vi "New File.vi"(8 "error in (no error)":errorcluster, 11 "Log in":refnum<class "Log.lvclass">) -> (0 "error out":errorcluster, 3 "Log out":refnum<class "Log.lvclass">)   [LabVIEW 2020, in "Log.lvclass"]
doc: "Starts a new file. Increments the file count, resets the line count and writes the header information into the file."
uses:
  Log.lvclass
  Log.lvclass/Log.ctl
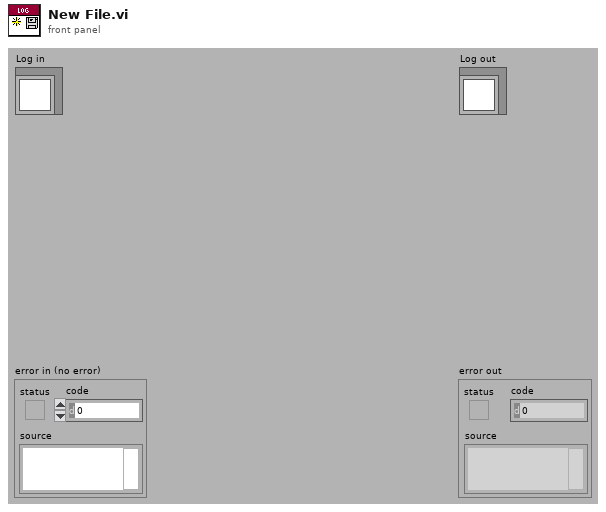
[diagram p1: front panel]
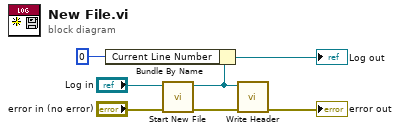
[diagram p0: block diagram]
diagram:
  n1 = call "Start New File.vi"("error in (no error)"="error in (no error)", "Log in"="Log in") -> ("error out"=w3:errorcluster, "Log out"=w1:refnum<class "Log.lvclass">)  [unwired: 8 out]
  n2 = Bundle By Name(cluster=w1, "Current Line Number"=0 ("Current Record")) -> (→"Log out":refnum<class "Log.lvclass">)
  n3 = call "Write Header.vi"("error in (no error)"=w3, "Log in"=w1) -> ("error out"=→"error out":errorcluster)  [unwired: 1 in, 8 out]
